vi "Param Read.vi"(4 "error in (no error)":errorcluster, 6 "Container State":T5, 7 "Display State In":T2={"param"=[], "positions"=[0.0, 0.0, 0.0], "CellsI"=enum."5", "CellsIII"=enum."7", "DLI short "=refnum, "DLIII short"=refnum, "DLII long"=refnum, "step,ps"=100, " preset pos"=[]}) -> (0 "error out":errorcluster, 2 "Value":T1, 3 "Display State Out":T2={"param"=[], "positions"=[0.0, 0.0, 0.0], "CellsI"=enum."5", "CellsIII"=enum."7", "DLI short "=refnum, "DLIII short"=refnum, "DLII long"=refnum, "step,ps"=100, " preset pos"=[]})   [LabVIEW 2019, in "ControlDL.xctl"]
uses:
  ControlDL.xctl
  <vilib>/_xctls/Container State.ctl
  <vilib>/_xctls/XControlSupport.lvlib
  stateDL.ctl
  controls/CellBoolean.ctl
  controls/CellsSDIII.ctl
  controls/CellsSDI.ctl
panel:
  # "Replace the Value Indicator below with an Indicator of desired type.\nDo not remove this Indicator or the others from the connector pane. \nDo not change the connector pane pattern.\nThe Value Indicator should always be the second terminal from top on the output side in the connector pane."
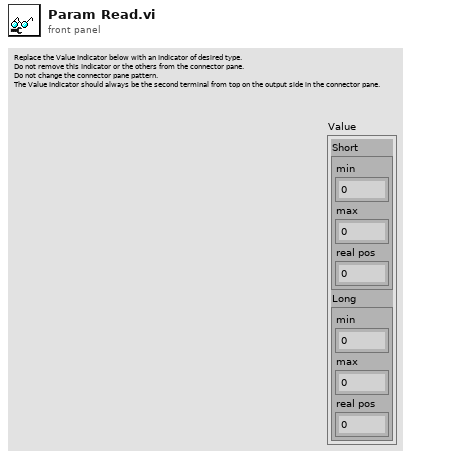
[diagram p1: front panel]
types:
  T1 = cluster{"Short":cluster{"min":dbl, "max":dbl, "real pos":dbl}, "Long":cluster{"min":dbl, "max":dbl, "real pos":dbl}}
  T2 = typedef "ControlDL.xctl/stateDL.ctl" = cluster{"param":cluster{"min":dbl, "max":dbl, "real pos":dbl}[], "positions":dbl[], "CellsI":T3, "CellsIII":T4, "DLI short ":refnum<user-event>, "DLIII short":refnum<user-event>, "DLII long":refnum<user-event>, "step,ps":i32, " preset pos":dbl[][]}
  T3 = typedef "CellsSDI.ctl" = enum32{"5", "4", "3", "2", "1", "L"}
  T4 = typedef "CellsSDIII.ctl" = enum32{"7", "6", "5", "4", "3", "2", "1", "L"}
  T5 = typedef "XControlSupport.lvlib/Container State.ctl" = cluster{"Indicator?":bool, "Run Mode?":bool, " Refnum":refnum<vi>}
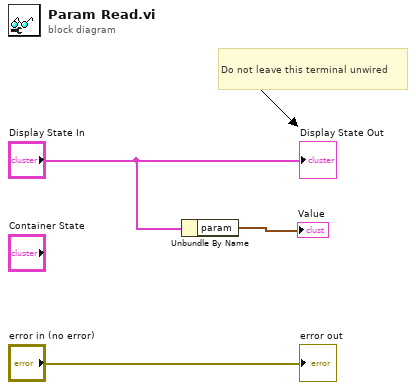
[diagram p0: block diagram]
diagram:
  # "Do not leave this terminal unwired"
  n1 = Unbundle By Name("Display State In") -> ("param"=→"Value":cluster{"min":dbl, "max":dbl, "real pos":dbl}[])
  "error out" <- "error in (no error)"
  "Display State Out" <- "Display State In"
